vi "Jog_104.vi"(0 "Axis_ID":i32, 1 "方向":bool, 3 "参数":cluster{"ACC":i32, "DEC":i32}, 4 "VM":i32, 5 "error in (no error)":errorcluster caption="错误输入（无错误）") -> (19 "error out":errorcluster caption="错误输出")   [LabVIEW 2017]
uses:
  APS168.lvlib
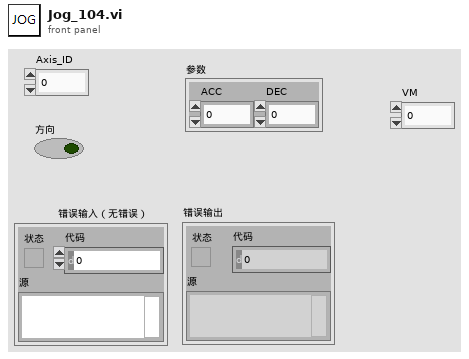
[diagram p1: front panel]
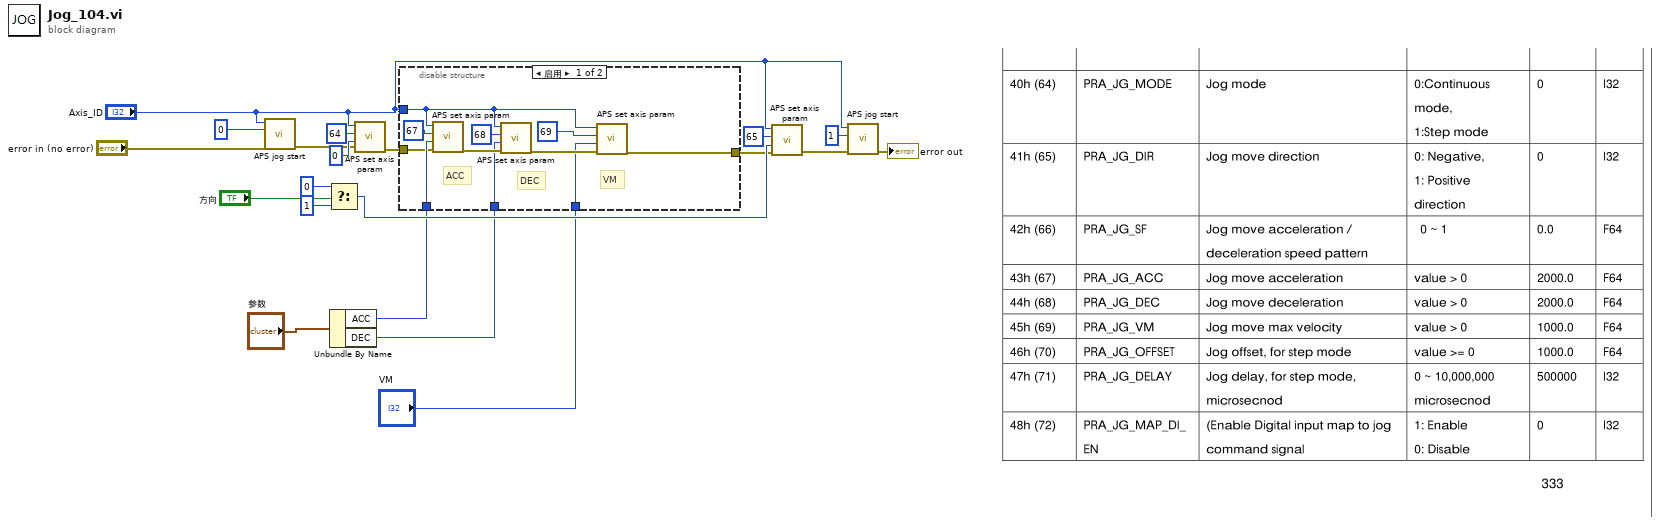
[diagram p0: block diagram]
diagram:
  n1 = call "APS jog start.vi"("error in (no error)"="error in (no error)", "On"=0, "Axis_ID"="Axis_ID") -> ("error out"=w1:errorcluster)  [unwired: 7 in, 1 out]
  n2 = Select(t=0, s="方向", f=1) -> (s? t:f=w16:i32)
  n3 = Unbundle By Name("参数") -> ("ACC"=w10:i32, "DEC"=w9:i32)
  n4 = call "APS set axis param.vi"("error in (no error)"=w1, "AXS_Param"=0, "AXS_Param_No"=64, "Axis_ID"="Axis_ID") -> ("error out"=w7:errorcluster)  [unwired: 6 in, 1 out]
  n5 = disable-structure shown="启用" {
    disable-tunnel: "Axis_ID" -> [w27 _]
    disable-tunnel: w10 -> [w25 _]
    disable-tunnel: w9 -> [w24 _]
    disable-tunnel: "VM" -> [w23 _]
    disable-tunnel: w7 -> [w22 w32]
    disable-tunnel: [w21 w32] -> w6
    frame Enabled {
      # "VM"
      # "DEC"
      # "ACC"
      n6 = call "APS set axis param.vi"("error in (no error)"=w22, "AXS_Param"=w25, "AXS_Param_No"=67, "Axis_ID"=w27) -> ("error out"=w30:errorcluster)  [unwired: 6 in, 1 out]
      n7 = call "APS set axis param.vi"("error in (no error)"=w30, "AXS_Param"=w24, "AXS_Param_No"=68, "Axis_ID"=w27) -> ("error out"=w28:errorcluster)  [unwired: 6 in, 1 out]
      n8 = call "APS set axis param.vi"("error in (no error)"=w28, "AXS_Param"=w23, "AXS_Param_No"=69, "Axis_ID"=w27) -> ("error out"=w21:errorcluster)  [unwired: 6 in, 1 out]
    }
    frame Disabled {
    }
  }
  n9 = call "APS set axis param.vi"("error in (no error)"=w6, "AXS_Param"=w16, "AXS_Param_No"=65, "Axis_ID"="Axis_ID") -> ("error out"=w5:errorcluster)  [unwired: 6 in, 1 out]
  n10 = call "APS jog start.vi"("error in (no error)"=w5, "On"=1, "Axis_ID"="Axis_ID") -> ("error out"=→"error out":errorcluster)  [unwired: 7 in, 1 out]
